vi "Process Order Item.vi"(8 "error in (no error)":errorcluster, 10 "Order Item.lvclass":refnum<class "Order Item.lvclass">, 11 "Barista in":refnum<class "Barista.lvclass">) -> (0 "error out":errorcluster, 3 "Barista out":refnum<class "Barista.lvclass">)   [LabVIEW 2020, in "Barista.lvclass"]
uses:
  Barista.lvclass
  C:/Users/anton/Documents/GitHub/Triarc-Examples/Coffee Shop/Person/Person.lvclass
  Support/Order Item/Order Item.lvclass
  Person/Person.lvclass
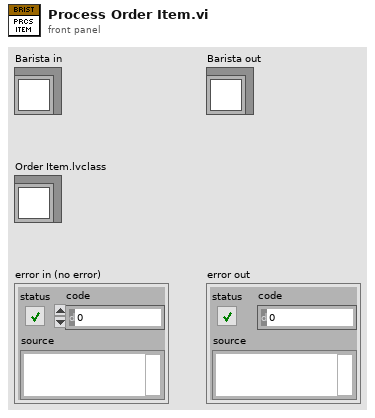
[diagram p1: front panel]
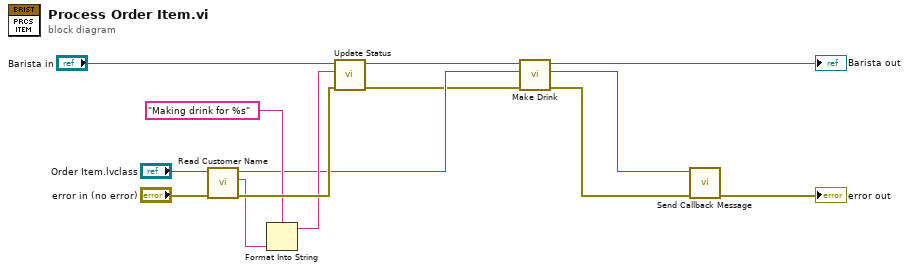
[diagram p0: block diagram]
diagram:
  n1 = call-dynamic "Read Customer Name.vi"("error in (no error)"="error in (no error)", "Order Item in"="Order Item.lvclass") -> ("error out"=w14:errorcluster, "Customer Name"=w11:string, "Order Item out"=w7:refnum<class "Order Item.lvclass">)  [unwired: 7 in]
  n2 = Format Into String(format string="Making drink for %s", w11) -> (resulting string=w13:string)  [unwired: 2 in, 1 out]
  n3 = call "Update Status.vi"("error in (no error)"=w14, "Status"=w13, "Person In"="Barista in") -> ("error out"=w6:errorcluster, "Person Out"=w3:refnum<class "Barista.lvclass">)  [unwired: 7 in]
  n4 = call "Make Drink.vi"("error in (no error)"=w6, "Order Item in"=w7, "Barista in"=w3) -> ("error out"=w5:errorcluster, "Order Item out"=w1:refnum<class "Order Item.lvclass">, "Barista out"=→"Barista out":refnum<class "Barista.lvclass">)  [unwired: 6 in]
  n5 = call-dynamic "Send Callback Message.vi"("error in (no error)"=w5, "Order Item in"=w1) -> ("error out"=→"error out":errorcluster)  [unwired: 8 in, 1 out]
